vi "Destroy.vi"(8 "error in (no error)":errorcluster, 11 "VariantAttribute in":refnum<class "MapImp.lvclass">) -> (0 "error out":errorcluster, 7 "VariantAttribute out":refnum<class "MapImp.lvclass">)   [LabVIEW 2013, in "LapDog.Collections.v1.Maps.lvlib" / "MapImp.lvclass"]
uses:
  MapImp.lvclass
  MapImp.lvclass/MapImp.ctl
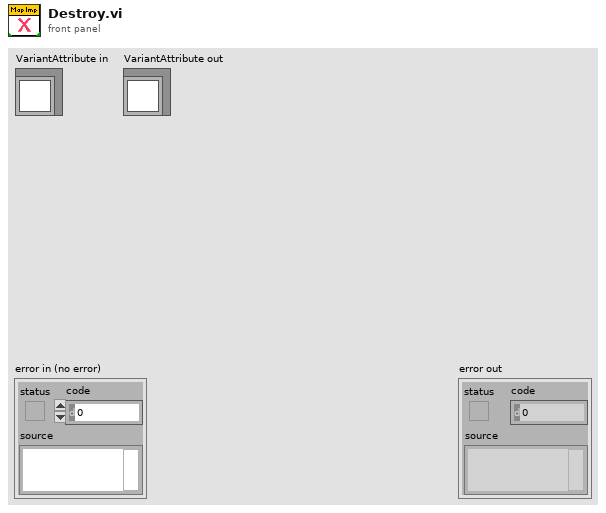
[diagram p1: front panel]
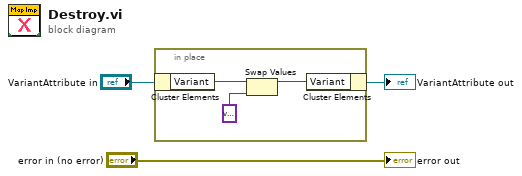
[diagram p0: block diagram]
diagram:
  n1 = in-place {
    n2 = in-place-cluster #1("VariantAttribute in") -> ("Variant"=w6:variant)
    n3 = Swap Values(12:w6, 14:variant) -> (1:w5:variant)  [unwired: 1 in, 1 out]
    n4 = in-place-cluster #1("Variant"=w5) -> (→"VariantAttribute out":refnum<class "MapImp.lvclass">)
  }
  "error out" <- "error in (no error)"
